vi "Read.vi"(11 "GroupsValue in":refnum<class "GroupNamesValue.lvclass">) -> (2 "Groups":string[](array[string]))   [LabVIEW 2020, in "Vecto.lvlib" / "GroupNamesValue.lvclass"]
uses:
  GroupNamesValue.lvclass
  GroupNamesValue.lvclass/GroupNamesValue.ctl
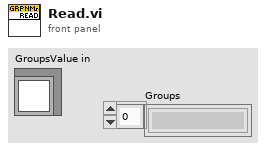
[diagram p1: front panel]
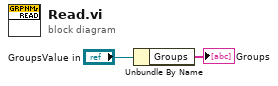
[diagram p0: block diagram]
diagram:
  n1 = Unbundle By Name("GroupsValue in") -> ("Groups"=→"Groups":string[])
